vi "LV2Creation_Script.vi"(8 "error in (no error)":errorcluster, 11 "SelList[]":refnum<vi>[](array[refnum])) -> (0 "error out":errorcluster)   [LabVIEW 2014]
uses:
  <vilib>/Utility/miscctls.llb/LVPointTypeDef.ctl
panel:
  out "Class Name":string
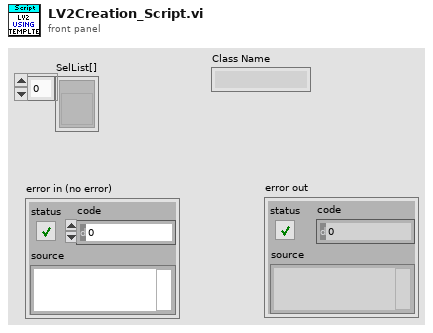
[diagram p1: front panel]
types:
  T1 = typedef "LVPointTypeDef.ctl" = cluster{"Horizontal":i16, "Vertical":i16}
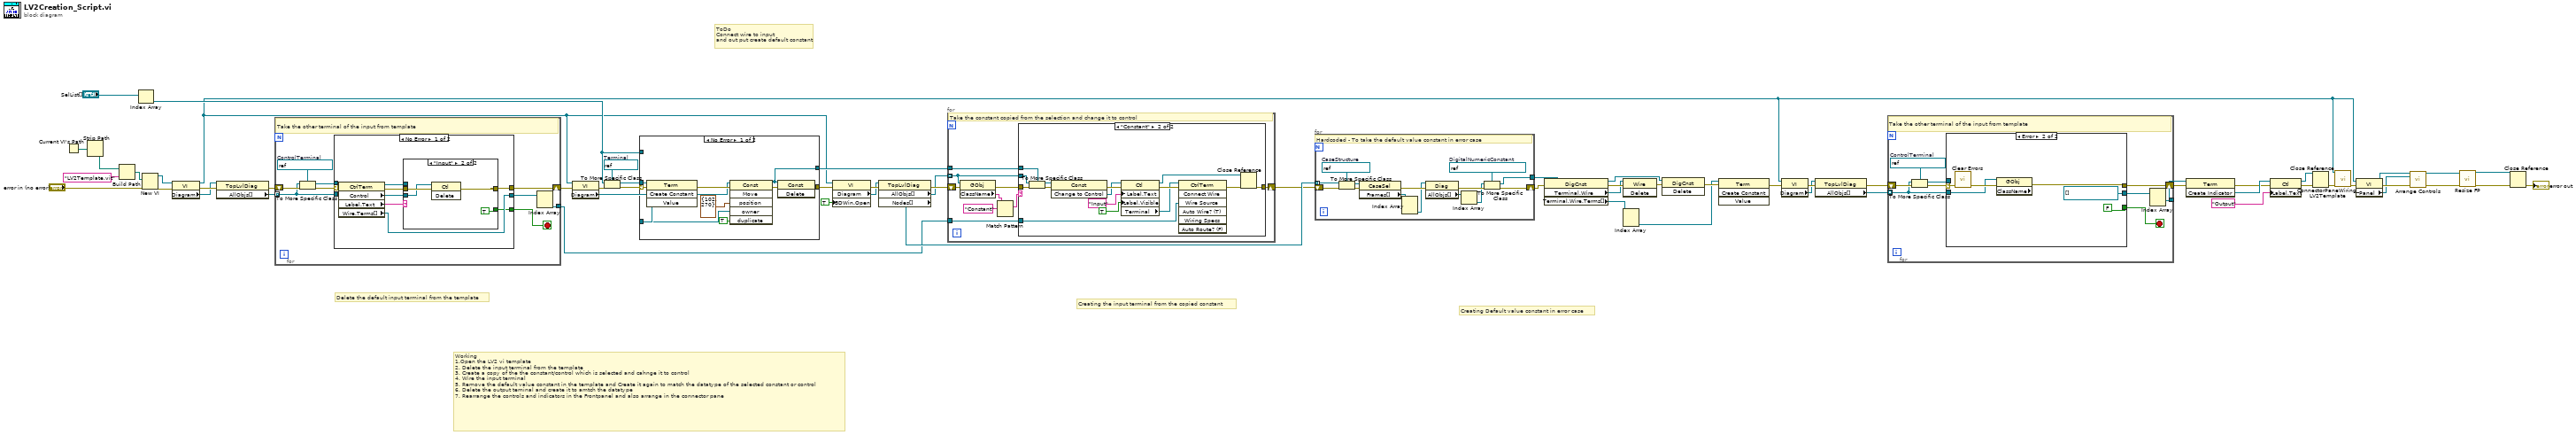
[diagram p0: block diagram]
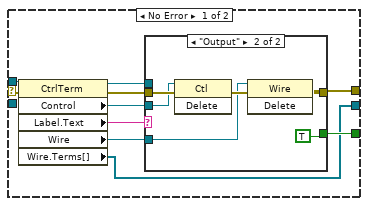
[diagram p2: hidden frame]
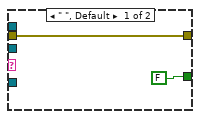
[diagram p3: hidden frame]
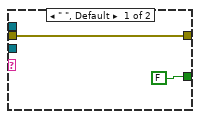
[diagram p4: hidden frame]
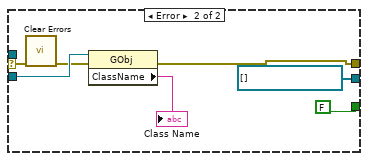
[diagram p5: hidden frame]
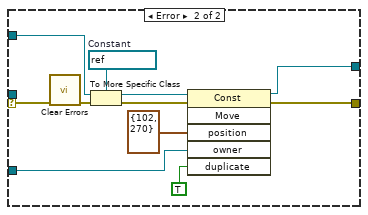
[diagram p7: hidden frame]
diagram:
  w60 = refnum<vi> refnum  # Terminal
  # "Working\n1.Open the LV2 vi template\n2. Delete the input terminal from the template\n3. Create a copy of the the constant/control which is selected and cahnge it to control\n4. Wire the input terminal\n5. Remove the default value constant in the template and Create it again to match the datatype of the selected constant or control\n6. Delete the output teminal and create it to amtch the datatype\n7. Rearrange the controls and indicators in the Frontpanel and also arrange in the connector pane"
  # "Delete the default input terminal from the template"
  # "Creating the input terminal from the copied constant"
  # "Creating Default value constant in error case"
  # "ToDo\nConnect wire to input\nand out put create default constant"
  n1 = Current VI's Path() -> (path=w46:path)
  n2 = Strip Path(path=w46) -> (stripped path=w43:path)  [unwired: 1 out]
  n3 = Build Path(base path=w43, name or relative path="LV2Template.vit") -> (appended path=w47:path)
  n4 = Index Array(array="SelList[]") -> (element=w57:refnum<vi>)  [unwired: 1 in]
  n5 = New VI(8:"error in (no error)", 10:w47) -> (0:w56:errorcluster, 3:w48:refnum<vi>)  [unwired: 5 in]
  n6 = property class="VI"(reference=w48, error in=w56) -> (reference out=w5:refnum<vi>, error out=w55:errorcluster, "Diagram"=w40:refnum<vi>)
  n7 = property class="TopLvlDiag"(reference=w40, error in=w55) -> (error out=w39:errorcluster, "AllObjs[]"=w38:refnum<vi>[])  [unwired: 1 out]
  n8 = for {
    shift-right: [w70] -> w36
    shift-left: w39 -> [w69]
    tunnel: w38 -> [w62] mode=indexing
    tunnel: [w63] -> w37
    stop <- w65 stop-if-true
    w68 = refnum<vi> refnum  # ControlTerminal
    # "Take the other terminal of the input from template"
    n9 = To More Specific Class(target class=w68, reference=w62, error in=w69) -> (specific class reference=w67:refnum<vi>, error out=w66:errorcluster)
    n10 = case shown="No Error" w66 {
      selector: w66 -> [w77 w92]
      tunnel: [w76 w89] -> w70
      tunnel: w67 -> [w78 _]
      tunnel: [w71 FALSE] -> w65
      tunnel: [w73 refnum<vi>[] [] ("Terminal.Wire.Terms[]")] -> w64
      tunnel: w62 -> [_ w88]
      frame No Error {
        n11 = property class="CtrlTerm"(reference=w78, error in=w77) -> (reference out=w75:refnum<vi>, error out=w79:errorcluster, "Control"=w72:refnum<vi>, "Label.Text"=w74:string, "Wire.Terms[]"=w73:refnum<vi>[])
        n12 = case shown="\"Input\"" w74 {
          tunnel: w79 -> [w81 w85]
          tunnel: [w81 w84] -> w76
          tunnel: w75 -> [_ _]
          tunnel: w72 -> [_ w83]
          tunnel: [FALSE TRUE] -> w71
          frame " ", Default {
          }
          frame "Input" {
            n13 = invoke class="Ctl" method="Delete"(reference=w83, error in=w85) -> (error out=w84:errorcluster)  [unwired: 1 in, 2 out]
          }
        }
      }
      frame Error {
        n14 = call <vilib>:"Clear Errors.vi"("error in (no error)"=w92) -> ("error out"=w86:errorcluster)  [unwired: 5 in, 1 out]
        n15 = property class="GObj"(reference=w88, error in=w86) -> (error out=w89:errorcluster, "ClassName"=→"Class Name":string)  [unwired: 1 out]
      }
    }
    n16 = Index Array(array=w64) -> (element #2=w63:refnum<vi>)  [unwired: 2 in, 1 out]
  }
  n17 = property class="VI"(reference=w5, error in=w36) -> (error out=w35:errorcluster, "Diagram"=w34:refnum<vi>)  [unwired: 1 out]
  n18 = To More Specific Class(target class=w60, reference=w57, error in=w35) -> (specific class reference=w59:refnum<vi>, error out=w58:errorcluster)
  n19 = case shown="No Error" w58 {
    selector: w58 -> [w97 w113]
    tunnel: w59 -> [w98 _]
    tunnel: [w94 w103] -> w54
    tunnel: w57 -> [_ w105]
    tunnel: w34 -> [w99 w106]
    tunnel: [w93 w104] -> w49
    frame No Error {
      n20 = invoke class="Term" method="Create Constant"(reference=w98, error in=w97) -> (error out=w102:errorcluster, "Create Constant"=w101:refnum<vi>)  [unwired: 2 in, 2 out]
      n21 = invoke class="Const" method="Move"(reference=w101, error in=w102, "position"=T1 {"Horizontal"=102, "Vertical"=270} ("location"), "owner"=w99, "duplicate"=TRUE ("Duplicate? (F)")) -> (reference out=w93:refnum<vi>, error out=w95:errorcluster)  [unwired: 1 in, 4 out]
      n22 = invoke class="Const" method="Delete"(reference=w93, error in=w95) -> (error out=w94:errorcluster)  [unwired: 1 in, 2 out]
    }
    frame Error {
      w111 = refnum<vi> refnum  # Constant
      n23 = call <vilib>:"Clear Errors.vi"("error in (no error)"=w113) -> ("error out"=w112:errorcluster)  [unwired: 5 in, 1 out]
      n24 = To More Specific Class(target class=w111, reference=w105, error in=w112) -> (specific class reference=w108:refnum<vi>, error out=w109:errorcluster)
      n25 = invoke class="Const" method="Move"(reference=w108, error in=w109, "position"=T1 {"Horizontal"=102, "Vertical"=270} ("location"), "owner"=w106, "duplicate"=TRUE ("Duplicate? (F)")) -> (reference out=w104:refnum<vi>, error out=w103:errorcluster)  [unwired: 1 in, 4 out]
    }
  }
  n26 = property class="VI"(reference=w5, error in=w54, "BDWin.Open"=TRUE ("Block Diagram Window:Open")) -> (error out=w53:errorcluster, "Diagram"=w42:refnum<vi>)  [unwired: 1 out]
  n27 = property class="TopLvlDiag"(reference=w42, error in=w53) -> (error out=w52:errorcluster, "AllObjs[]"=w51:refnum<vi>[], "Nodes[]"=w41:refnum<vi>[])  [unwired: 1 out]
  n28 = for {
    tunnel: w51 -> [w119] mode=indexing
    tunnel: w49 -> [w121]
    shift-right: [w118] -> w24
    shift-left: w52 -> [w122]
    tunnel: w37 -> [w114]
    # "Take the constant copied from the selection and change it to control"
    n29 = property class="GObj"(reference=w119, error in=w122) -> (error out=w120:errorcluster, "ClassName"=w116:string)  [unwired: 1 out]
    n30 = Match Pattern(string=w116, regular expression="Constant") -> (match substring=w115:string)  [unwired: 1 in, 3 out]
    n31 = case shown="\"Constant\"" w115 {
      tunnel: w120 -> [w123 w138]
      tunnel: w119 -> [_ w137]
      tunnel: w121 -> [_ w134]
      tunnel: [w123 w128] -> w118
      tunnel: w114 -> [_ w124]
      frame " ", Default {
      }
      frame "Constant" {
        n32 = To More Specific Class(target class=w134, reference=w137, error in=w138) -> (specific class reference=w135:refnum<vi>, error out=w136:errorcluster)
        n33 = invoke class="Const" method="Change to Control"(reference=w135, error in=w136) -> (error out=w131:errorcluster, "Change to Control"=w129:refnum<vi>)  [unwired: 1 in, 1 out]
        n34 = property class="Ctl"(reference=w129, error in=w131, "Label.Text"="Input", "Label.Visible"=TRUE) -> (reference out=w125:refnum<vi>, error out=w130:errorcluster, "Terminal"=w126:refnum<vi>)
        n35 = invoke class="CtrlTerm" method="Connect Wire"(reference=w126, error in=w130, "Wire Source"=w124) -> (error out=w127:errorcluster)  [unwired: 4 in, 6 out]
        n36 = Close Reference(reference=w125, error in (no error)=w127) -> (error out=w128:errorcluster)
      }
    }
  }
  n37 = for {
    tunnel: w41 -> [w150] mode=indexing
    tunnel: [w141] -> w32
    shift-right: [w140] -> w25
    shift-left: w24 -> [w139]
    w142 = refnum<vi> refnum  # DigitalNumericConstant
    w148 = refnum<vi> refnum  # CaseStructure
    # "Hardcoded - To take the default value constant in error case"
    n38 = To More Specific Class(target class=w148, reference=w150, error in=w139) -> (specific class reference=w149:refnum<vi>, error out=w151:errorcluster)
    n39 = property class="CaseSel"(reference=w149, error in=w151) -> (error out=w152:errorcluster, "Frames[]"=w147:refnum<vi>[])  [unwired: 1 out]
    n40 = Index Array(array=w147) -> (element #2=w145:refnum<vi>)  [unwired: 2 in, 1 out]
    n41 = property class="Diag"(reference=w145, error in=w152) -> (error out=w144:errorcluster, "AllObjs[]"=w146:refnum<vi>[])  [unwired: 1 out]
    n42 = Index Array(array=w146) -> (element=w143:refnum<vi>)  [unwired: 1 in]
    n43 = To More Specific Class(target class=w142, reference=w143, error in=w144) -> (specific class reference=w141:refnum<vi>, error out=w140:errorcluster)
  }
  n44 = property class="DigCnst"(reference=w32, error in=w25) -> (reference out=w29:refnum<vi>, error out=w33:errorcluster, "Terminal.Wire"=w30:refnum<vi>, "Terminal.Wire.Terms[]"=w31:refnum<vi>[])
  n45 = invoke class="Wire" method="Delete"(reference=w30, error in=w33) -> (error out=w28:errorcluster)  [unwired: 1 in, 2 out]
  n46 = Index Array(array=w31) -> (element #2=w26:refnum<vi>)  [unwired: 2 in, 1 out]
  n47 = invoke class="DigCnst" method="Delete"(reference=w29, error in=w28) -> (error out=w27:errorcluster)  [unwired: 1 in, 2 out]
  n48 = invoke class="Term" method="Create Constant"(reference=w26, error in=w27) -> (error out=w23:errorcluster)  [unwired: 2 in, 3 out]
  n49 = property class="VI"(reference=w5, error in=w23) -> (error out=w21:errorcluster, "Diagram"=w6:refnum<vi>)  [unwired: 1 out]
  n50 = property class="TopLvlDiag"(reference=w6, error in=w21) -> (error out=w20:errorcluster, "AllObjs[]"=w19:refnum<vi>[])  [unwired: 1 out]
  n51 = for {
    shift-right: [w161] -> w22
    shift-left: w20 -> [w160]
    tunnel: w19 -> [w154] mode=indexing
    tunnel: [w153] -> w18
    stop <- w156 stop-if-true
    w159 = refnum<vi> refnum  # ControlTerminal
    # "Take the other terminal of the input from template"
    n52 = To More Specific Class(target class=w159, reference=w154, error in=w160) -> (specific class reference=w158:refnum<vi>, error out=w157:errorcluster)
    n53 = case shown="Error" w157 {
      selector: w157 -> [w169 w185]
      tunnel: [w168 w181] -> w161
      tunnel: w158 -> [w170 _]
      tunnel: [w164 FALSE] -> w156
      tunnel: [w163 refnum<vi>[] [] ("Terminal.Wire.Terms[]")] -> w155
      tunnel: w154 -> [_ w180]
      frame No Error {
        n54 = property class="CtrlTerm"(reference=w170, error in=w169) -> (reference out=w167:refnum<vi>, error out=w171:errorcluster, "Control"=w165:refnum<vi>, "Label.Text"=w166:string, "Wire"=w162:refnum<vi>, "Wire.Terms[]"=w163:refnum<vi>[])
        n55 = case shown="\"Output\"" w166 {
          tunnel: w171 -> [w173 w179]
          tunnel: [w173 w175] -> w168
          tunnel: w167 -> [_ _]
          tunnel: w165 -> [_ w178]
          tunnel: [FALSE TRUE] -> w164
          tunnel: w162 -> [_ w174]
          frame " ", Default {
          }
          frame "Output" {
            n56 = invoke class="Ctl" method="Delete"(reference=w178, error in=w179) -> (error out=w176:errorcluster)  [unwired: 1 in, 2 out]
            n57 = invoke class="Wire" method="Delete"(reference=w174, error in=w176) -> (error out=w175:errorcluster)  [unwired: 1 in, 2 out]
          }
        }
      }
      frame Error {
        n58 = call <vilib>:"Clear Errors.vi"("error in (no error)"=w185) -> ("error out"=w182:errorcluster)  [unwired: 5 in, 1 out]
        n59 = property class="GObj" props=["ClassName"](reference=w180, error in=w182) -> (error out=w181:errorcluster)  [unwired: 2 out]
      }
    }
    n60 = Index Array(array=w155) -> (element #1=w153:refnum<vi>)  [unwired: 2 in, 1 out]
  }
  n61 = invoke class="Term" method="Create Indicator"(reference=w18, error in=w22) -> (error out=w13:errorcluster, "Create Indicator"=w17:refnum<vi>)  [unwired: 1 in, 1 out]
  n62 = property class="Ctl"(reference=w17, error in=w13, "Label.Text"="Output") -> (reference out=w14:refnum<vi>, error out=w15:errorcluster)
  n63 = Close Reference(reference=w14, error in (no error)=w15) -> (error out=w8:errorcluster)
  n64 = call "ConnectorPaneWiring_LV2Template.vi"("VI in"=w5, "error in (no error)"=w8) -> ("error out"=w7:errorcluster)  [unwired: 13 in]
  n65 = property class="VI"(reference=w5, error in=w7) -> (reference out=w10:refnum<vi>, error out=w12:errorcluster, "Panel"=w11:refnum<vi>)
  n66 = call "Arrange Controls.vi"("VI in"=w10, "front panel"=w11, "error in"=w12) -> ("VI out"=w2:refnum<vi>, "error out"=w4:errorcluster)  [unwired: 11 in]
  n67 = call "Resize FP.vi"("VI in"=w2, "error in"=w4) -> ("VI out"=w1:refnum<vi>, "error out"=w3:errorcluster)  [unwired: 12 in]
  n68 = Close Reference(reference=w1, error in (no error)=w3) -> (error out=→"error out":errorcluster)
